vi "Panel Split Example.vi"(10 "Caller":string) -> ()   [LabVIEW 2013]
uses:
  PanelRootNode/PanelRootNode.lvclass
  <vilib>/Utility/error.llb/DialogType.ctl
  PanelExample.lvclass
  share/QueueManager.llb/Destroy.vi
  share/QueueManager.llb/CreatQueue.vi
  share/QueueManager.llb/Remove.vi
  PanelLinkNode/PanelLinkNode.lvclass
  PanelDataNode/PanelDataNode.lvclass
panel:
  out "SelfNode*":refnum<data-value>
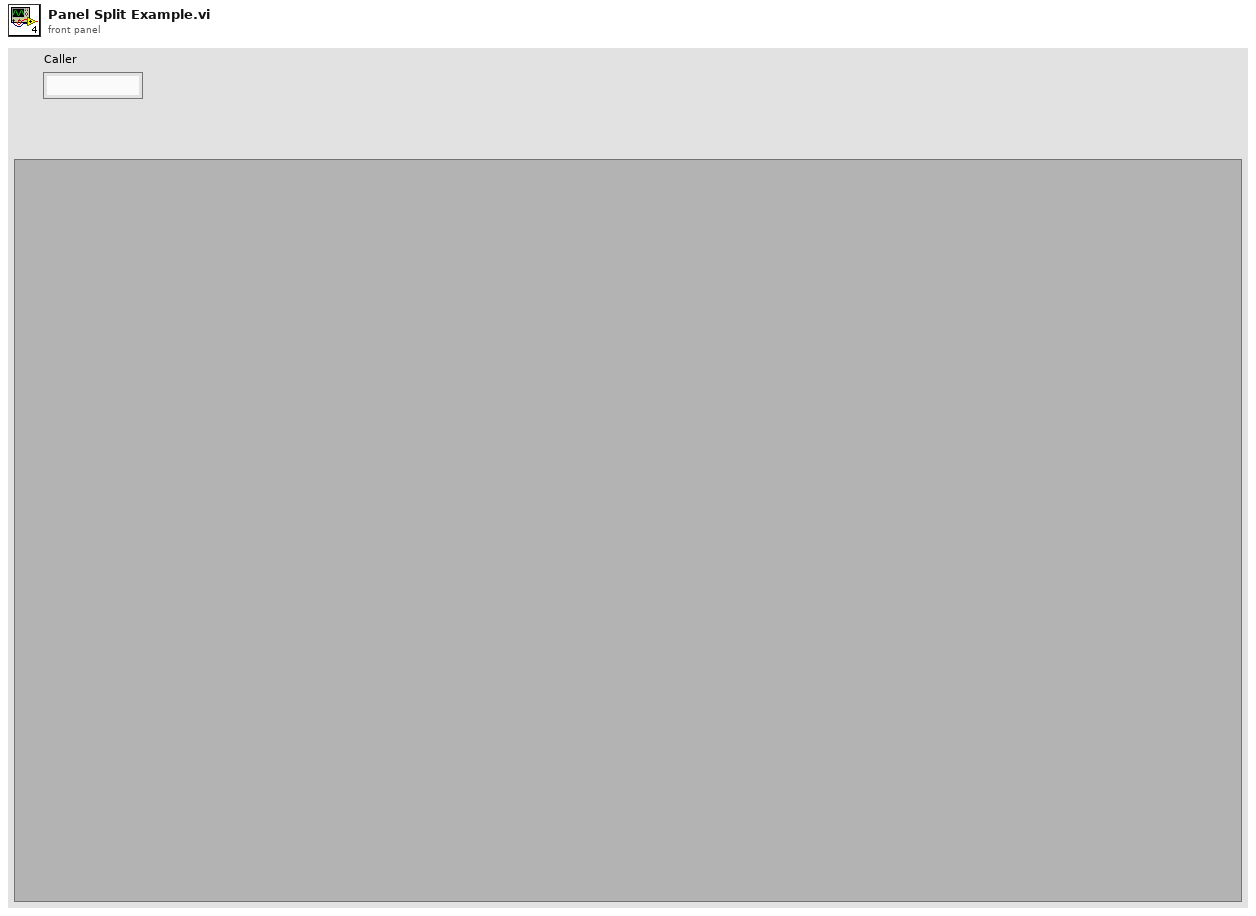
[diagram p1: front panel]
types:
  T1 = cluster{"error":errorcluster, "Event":string, "Data":variant, "Q_Local":string, "RootNode*":refnum<data-value>, "Caller":string}
  T2 = typedef "DialogType.ctl" = u16
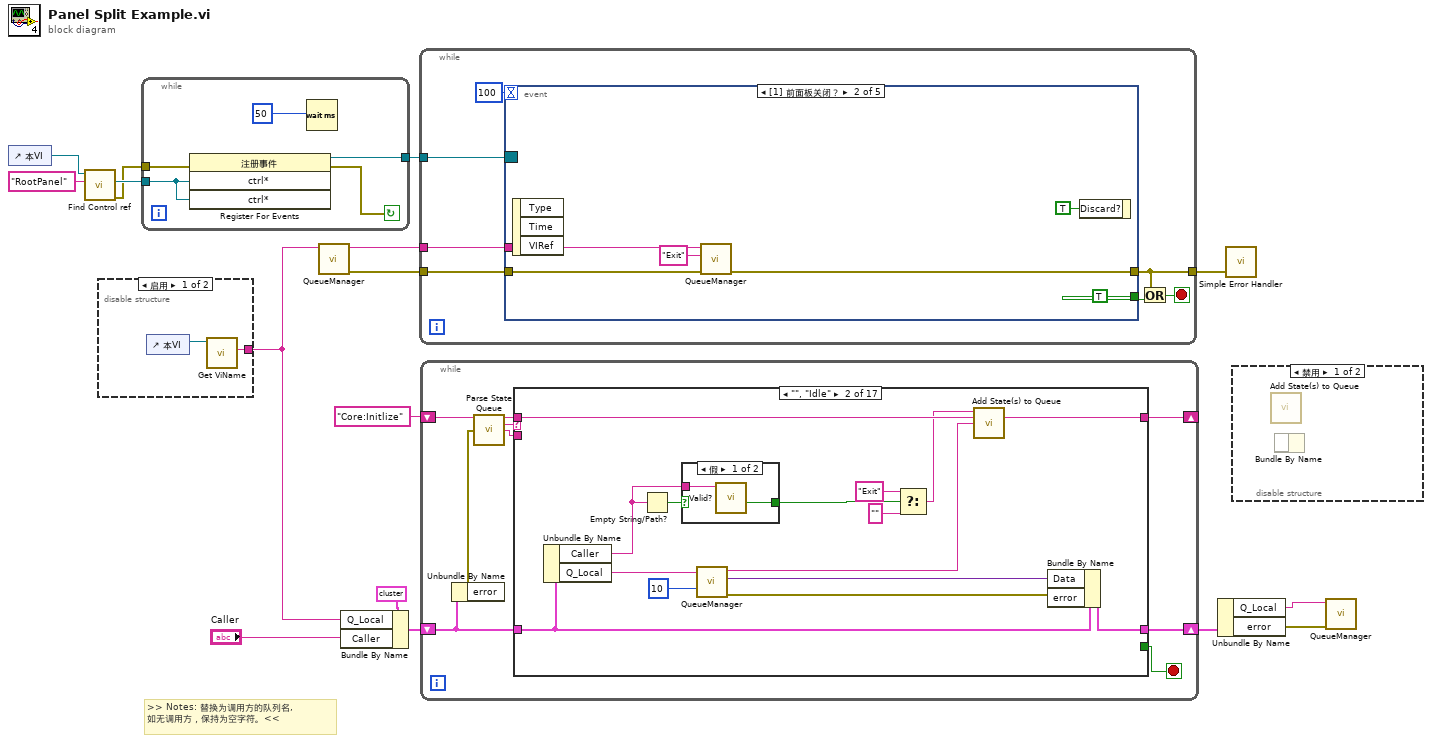
[diagram p0: block diagram]
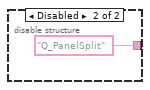
[diagram p2: hidden frame]
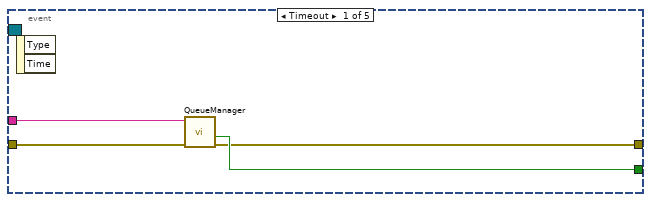
[diagram p4: hidden frame]
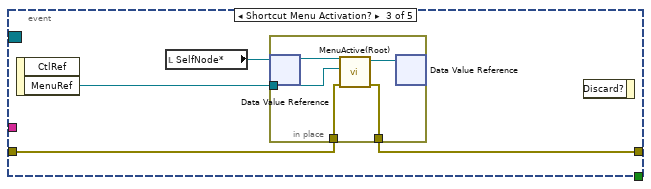
[diagram p5: hidden frame]
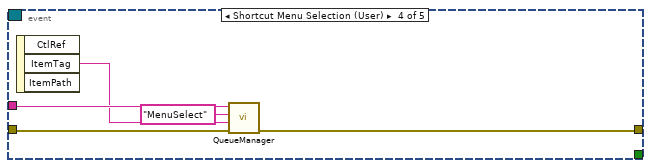
[diagram p6: hidden frame]
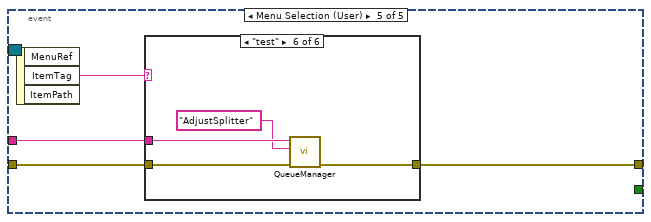
[diagram p7: hidden frame]
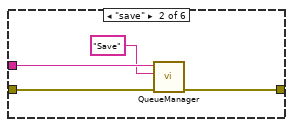
[diagram p9: hidden frame]
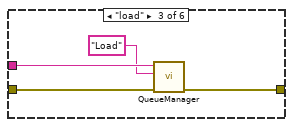
[diagram p10: hidden frame]
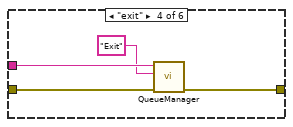
[diagram p11: hidden frame]
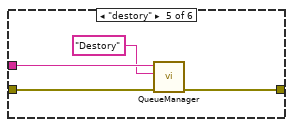
[diagram p12: hidden frame]
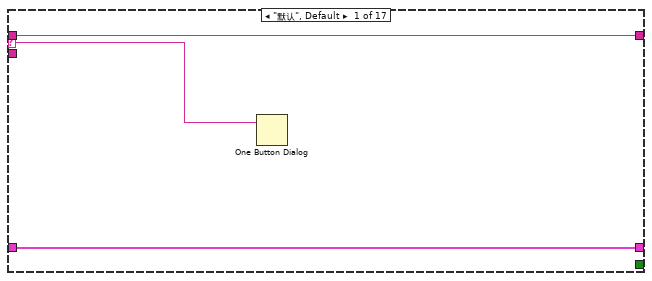
[diagram p13: hidden frame]
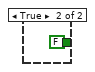
[diagram p14: hidden frame]
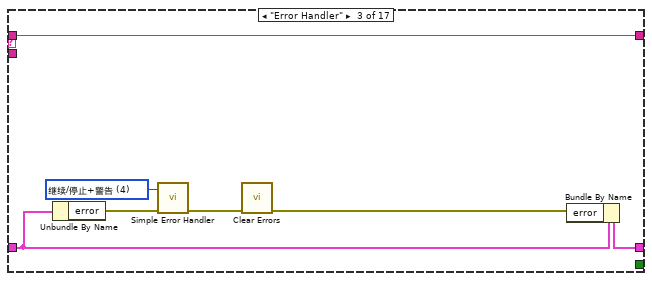
[diagram p15: hidden frame]
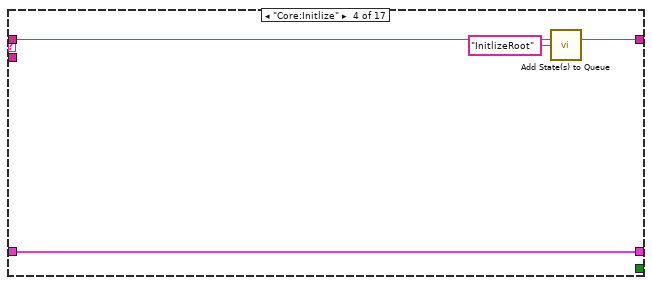
[diagram p16: hidden frame]
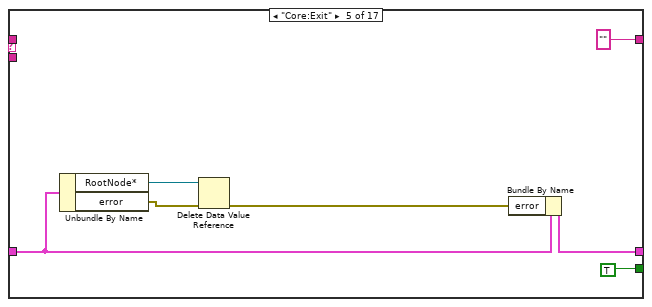
[diagram p17: hidden frame]
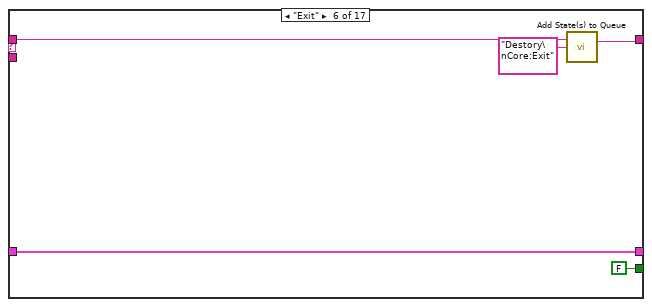
[diagram p18: hidden frame]
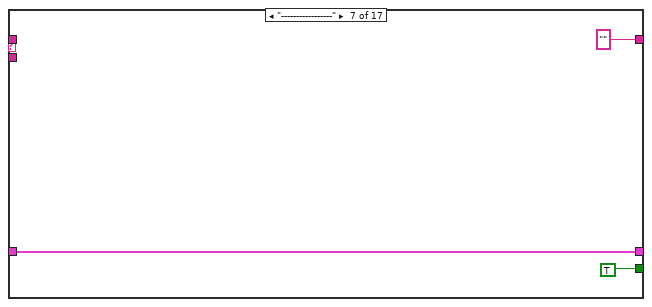
[diagram p19: hidden frame]
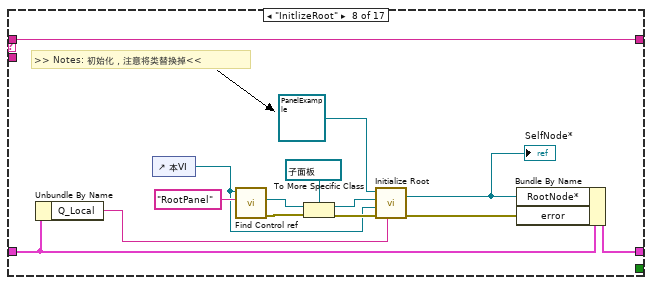
[diagram p20: hidden frame]
diagram:
  # ">> Notes: 替换为调用方的队列名,\n如无调用方，保持为空字符。<<"
  n1 = control-ref of="本VI"() -> (w7:refnum<vi>)
  n2 = call "Find Control ref.vi"("control name"="RootPanel", "panelvi*"=w7) -> ("error out"=w2:errorcluster, "ctrl*"=w5:refnum<vi>)  [unwired: 7 in, 1 out]
  n3 = disable-structure shown="启用" {
    disable-tunnel: [w16 "Q_PanelSplit" ("QueueName")] -> w3
    frame Enabled {
      n4 = control-ref of="本VI"() -> (w17:refnum<vi>)
      n5 = call "Get ViName.vi"("VI*"=w17) -> ("VI Name"=w16:string)  [unwired: 8 in, 2 out]
    }
    frame Disabled {
    }
  }
  n6 = while {
    tunnel: w5 -> [w23]
    tunnel: [w22] -> w4
    tunnel: w2 -> [w21]
    stop <- w20 continue-if-true
    n7 = register-events(error in=w21, w23, w23) -> (reference out=w22:refnum<event-registration>, error out=w20:errorcluster)  [unwired: 1 in]
    n8 = Wait (ms)(milliseconds to wait=50) -> ()  [unwired: 1 out]
  }
  n9 = call-poly "QueueManager.vi"("QueueName"=w3) -> ("error out"=w15:errorcluster)  [unwired: 10 in]
  n10 = Bundle By Name(cluster=T1 {"error"={"status"=FALSE, "code"=0, "source"=""}, "Event"="", "Data"=variant, "Q_Local"="", "RootNode*"=refnum, "Caller"=""} ("TmpData"), "Q_Local"=w3, "Caller"="Caller") -> (w9:T1)
  n11 = while {
    tunnel: w15 -> [w29]
    tunnel: w3 -> [w30]
    tunnel: [w26] -> w11
    tunnel: w4 -> [w24]
    stop <- w27 stop-if-true
    n12 = event shown="[1] 前面板关闭？" {
      selector: w24 -> [_ _ _ _ _]
      dyn-events: _ -> [_ _ _ _ _]
      timeout: 100 -> [_ _ _ _ _]
      tunnel: [w32 TRUE _ _ _] -> w28
      tunnel: w30 -> [w34 w39 _ w54 w57]
      tunnel: w29 -> [w33 w38 w43 w53 w56]
      tunnel: [w31 w37 w44 w52 w55] -> w26
      event Timeout {
        n13 = event-data() -> ()  [unwired: 1 in, 2 out]
        n14 = call-poly "QueueManager.vi"("error in (no error)"=w33, "Queue Name(unamed)"=w34) -> ("error out"=w31:errorcluster, "Not Exist?"=w32:bool)  [unwired: 8 in]
      }
      event Panel Close? {
        n15 = event-data() -> ()  [unwired: 1 in, 3 out]
        n16 = call-poly "QueueManager.vi"("error in"=w38, "Event"="Exit", "QueueName"=w39) -> ("error out"=w37:errorcluster)  [unwired: 7 in, 1 out]
        n17 = event-data("Discard?"=TRUE ("放弃？")) -> ()  [unwired: 1 in, 1 out]
      }
      event Shortcut Menu Activation? {
        n18 = event-data() -> ("MenuRef"=w42:refnum<k9>)  [unwired: 1 in, 1 out]
        n19 = local read "SelfNode*"() -> (w41:refnum<data-value>)
        n20 = in-place {
          in-place-border: w42 -> [w47]
          in-place-border: w43 -> [w46]
          in-place-border: [w45] -> w44
          n21 = in-place-dvr #1(w41) -> (w49:refnum<class "PanelRootNode.lvclass">)  [unwired: 1 out]
          n22 = call "MenuActive(Root).vi"("error in (no error)"=w46, "菜单引用"=w47, "PanelDataNode 输入"=w49) -> ("error out"=w45:errorcluster, "PanelDataNode 输出"=w48:refnum<class "PanelRootNode.lvclass">)  [unwired: 7 in]
          n23 = in-place-dvr #1(w48) -> ()  [unwired: 2 out]
        }
        n24 = event-data() -> ()  [unwired: 2 in, 1 out]
      }
      event Shortcut Menu Selection (User) {
        n25 = event-data() -> ("ItemTag"=w51:string)  [unwired: 1 in, 2 out]
        n26 = call-poly "QueueManager.vi"("error in"=w53, "Data"=w51, "Event"="MenuSelect", "QueueName"=w54) -> ("error out"=w52:errorcluster)  [unwired: 6 in, 1 out]
      }
      event Menu Selection (User) {
        n27 = event-data() -> ("ItemTag"=w58:string)  [unwired: 1 in, 2 out]
        n28 = case shown="\"test\"" w58 {
          tunnel: w57 -> [_ w63 w67 w71 w75 w79]
          tunnel: w56 -> [w59 w61 w65 w69 w73 w77]
          tunnel: [w59 w60 w64 w68 w72 w76] -> w55
          frame "假", Default {
          }
          frame "save" {
            n29 = call-poly "QueueManager.vi"("error in"=w61, "Event"="Save", "QueueName"=w63) -> ("error out"=w60:errorcluster)  [unwired: 7 in, 1 out]
          }
          frame "load" {
            n30 = call-poly "QueueManager.vi"("error in"=w65, "Event"="Load", "QueueName"=w67) -> ("error out"=w64:errorcluster)  [unwired: 7 in, 1 out]
          }
          frame "exit" {
            n31 = call-poly "QueueManager.vi"("error in"=w69, "Event"="Exit", "QueueName"=w71) -> ("error out"=w68:errorcluster)  [unwired: 7 in, 1 out]
          }
          frame "destory" {
            n32 = call-poly "QueueManager.vi"("error in"=w73, "Event"="Destory", "QueueName"=w75) -> ("error out"=w72:errorcluster)  [unwired: 7 in, 1 out]
          }
          frame "test" {
            n33 = call-poly "QueueManager.vi"("error in"=w77, "Event"="AdjustSplitter", "QueueName"=w79) -> ("error out"=w76:errorcluster)  [unwired: 7 in, 1 out]
          }
        }
      }
    }
    n34 = Or(x=w26, y=w28) -> (x .or. y?=w27:bool)
  }
  n35 = while {
    shift-right: [w81] -> w12
    shift-left: w9 -> [w82]
    shift-right: [w80] -> _
    shift-left: "Core:Initlize" -> [w88]
    stop <- w84 stop-if-true
    n36 = Unbundle By Name(w82) -> ("error"=w83:errorcluster)
    n37 = call "Parse State Queue.vi"("State Queue"=w88, "Error In (no error)"=w83) -> ("Remaining States"=w87:string, "Current State"=w86:string, "Arguments"=w85:string)  [unwired: 10 in, 1 out]
    n38 = case shown="\"\", \"Idle\"" w86 {
      selector: w86 -> [w89 _ _ _ _ _ _ _ _ _ _ _ _ _ _ _ _]
      tunnel: w87 -> [w90 w102 w116 w119 _ w132 _ w149 w155 w171 w181 w196 w206 w216 w226 w235 w250]
      tunnel: w85 -> [_ _ _ _ _ _ _ _ _ _ _ _ _ _ _ _ _]
      tunnel: [_ _ _ _ TRUE FALSE TRUE _ _ _ _ _ _ _ _ _ _] -> w84
      tunnel: w82 -> [w91 w99 w112 w120 w123 w129 w134 w138 w157 w169 w185 w195 w204 w214 w224 w233 w248]
      tunnel: [w91 w105 w111 w120 w122 w129 w134 w141 w156 w168 w184 w194 w203 w213 w223 w232 w247] -> w81
      tunnel: [w90 w101 w116 w118 "" ("Remaining States") w131 "" ("Remaining States") w149 w155 w171 w180 w196 w206 w216 w226 w235 w250] -> w80
      frame "默认", Default {
        n39 = One Button Dialog(message=w89) -> ()  [unwired: 1 in, 1 out]
      }
      frame "", "Idle" {
        n40 = Unbundle By Name(w99) -> ("Caller"=w93:string, "Q_Local"=w98:string)
        n41 = Empty String/Path?(string/path=w93) -> (empty?=w97:bool)
        n42 = case shown="假" w97 {
          tunnel: [w108 FALSE ("Not Exist?")] -> w96
          tunnel: w93 -> [w107 _]
          frame False {
            n43 = call "Valid?.vi"("Queue Name(unamed)"=w107) -> ("Not Exist?"=w108:bool)  [unwired: 9 in, 1 out]
          }
          frame True {
          }
        }
        n44 = call-poly "QueueManager.vi"("Time out(-1)"=10, "Queue Name"=w98) -> ("error out"=w106:errorcluster, "Data"=w104:variant, "Event"=w103:string)  [unwired: 6 in, 1 out]
        n45 = Select(t="Exit" ("Event"), s=w96, f="") -> (s? t:f=w92:string)
        n46 = call "Add State(s) to Queue.vi"("State(s) in Front (\"\")"=w92, "State(s) in (\"\")"=w102, "State(s) at Back (\"\")"=w103) -> ("States Out"=w101:string)  [unwired: 12 in]
        n47 = Bundle By Name(cluster=w99, "Data"=w104, "error"=w106) -> (w105:T1)
      }
      frame "Error Handler" {
        w110 = T2 4 items=["无对话框", "确定信息", "继续或停止信息", "确定信息＋警告", "继续/停止+警告"] ("type of dialog (OK msg:1)")
        n48 = Unbundle By Name(w112) -> ("error"=w113:errorcluster)
        n49 = call <vilib>:"Simple Error Handler.vi"("type of dialog (OK msg:1)"=w110, "error in (no error)"=w113) -> ("error out"=w114:errorcluster)  [unwired: 3 in, 4 out]
        n50 = call <vilib>:"Clear Errors.vi"("error in (no error)"=w114) -> ("error out"=w115:errorcluster)  [unwired: 6 in]
        n51 = Bundle By Name(cluster=w112, "error"=w115) -> (w111:T1)
      }
      frame "Core:Initlize" {
        n52 = call "Add State(s) to Queue.vi"("State(s) in (\"\")"=w119, "State(s) at Back (\"\")"="InitlizeRoot" ("State(s) at Back (\"\")")) -> ("States Out"=w118:string)  [unwired: 13 in]
      }
      frame "Core:Exit" {
        n53 = Unbundle By Name(w123) -> ("RootNode*"=w125:refnum<data-value>, "error"=w121:errorcluster)
        n54 = Delete Data Value Reference(data value reference=w125, error in=w121) -> (error out=w124:errorcluster)  [unwired: 1 out]
        n55 = Bundle By Name(cluster=w123, "error"=w124) -> (w122:T1)
      }
      frame "Exit" {
        n56 = call "Add State(s) to Queue.vi"("State(s) in (\"\")"=w132, "State(s) at Back (\"\")"="Destory\nCore:Exit" ("State(s) at Back (\"\")")) -> ("States Out"=w131:string)  [unwired: 13 in]
      }
      frame "-----------------" {
      }
      frame "InitlizeRoot" {
        # ">> Notes: 初始化，注意将类替换掉<<"
        n57 = Unbundle By Name(w138) -> ("Q_Local"=w137:string)
        n58 = control-ref of="本VI"() -> (w139:refnum<vi>)
        n59 = call "Find Control ref.vi"("control name"="RootPanel", "panelvi*"=w139) -> ("error out"=w144:errorcluster, "ctrl*"=w148:refnum<vi>)  [unwired: 7 in, 1 out]
        n60 = To More Specific Class(target class=refnum<vi> refnum ("RootPanel"), reference=w148, error in=w144) -> (specific class reference=w146:refnum<vi>, error out=w143:errorcluster)
        n61 = call-dynamic "Initialize Root.vi"("RootQueueName"=w137, "error in (no error)"=w143, "CurrentVi*"=w139, "RootPanel*"=w146, "PanelRootNode 输入"=refnum<class "PanelExample.lvclass"> refnum ("PanelExample.lvclass")) -> ("error out"=w142:errorcluster, "SelfNode*"=w140:refnum<data-value>)  [unwired: 5 in]
        "SelfNode*" <- w140
        n62 = Bundle By Name(cluster=w138, "RootNode*"=w140, "error"=w142) -> (w141:T1)
      }
      frame "Save" {
        # ">> Notes: 保存分割结果<<"
        n63 = Unbundle By Name(w157) -> ("RootNode*"=w158:refnum<data-value>, "Data"=w153:variant)
        n64 = Variant To Data(type=path "" ("路径"), Variant=w153) -> (data=w151:path, error out=w150:errorcluster)  [unwired: 1 in]
        n65 = call <vilib>:"Clear Errors.vi"("error in (no error)"=w150) -> ()  [unwired: 6 in, 1 out]
        n66 = in-place {
          in-place-border: [w160] -> w154
          in-place-border: w151 -> [w159]
          n67 = in-place-dvr #2(w158) -> (w162:refnum<class "PanelRootNode.lvclass">)  [unwired: 1 out]
          n68 = call-dynamic "Save Xml.vi"("selected path"=w159, "PanelRootNode 输入"=w162) -> ("error out"=w160:errorcluster, "PanelRootNode 输出"=w161:refnum<class "PanelRootNode.lvclass">)  [unwired: 8 in]
          n69 = in-place-dvr #2(w161) -> ()  [unwired: 2 out]
        }
        n70 = Bundle By Name(cluster=w157, "error"=w154) -> (w156:T1)
      }
      frame "Load" {
        n71 = Unbundle By Name(w169) -> ("RootNode*"=w170:refnum<data-value>, "Data"=w164:variant)
        n72 = Variant To Data(type=path "" ("路径"), Variant=w164) -> (data=w163:path, error out=w165:errorcluster)  [unwired: 1 in]
        n73 = call <vilib>:"Clear Errors.vi"("error in (no error)"=w165) -> ()  [unwired: 6 in, 1 out]
        n74 = in-place {
          in-place-border: [w174] -> w167
          in-place-border: w163 -> [w172]
          n75 = in-place-dvr #3(w170) -> (w173:refnum<class "PanelRootNode.lvclass">)  [unwired: 1 out]
          n76 = call-dynamic "Load Xml.vi"("selected path"=w172, "PanelRootNode 输入"=w173) -> ("error out"=w174:errorcluster, "PanelRootNode 输出"=w175:refnum<class "PanelRootNode.lvclass">)  [unwired: 8 in]
          n77 = in-place-dvr #3(w175) -> ()  [unwired: 2 out]
        }
        n78 = Bundle By Name(cluster=w169, "error"=w167) -> (w168:T1)
      }
      frame "MenuSelect" {
        n79 = Unbundle By Name(w185) -> ("RootNode*"=w179:refnum<data-value>, "Data"=w183:variant)
        n80 = Variant To Data(type="", Variant=w183) -> (data=w178:string, error out=w177:errorcluster)  [unwired: 1 in]
        n81 = in-place {
          in-place-border: w178 -> [w188]
          in-place-border: w177 -> [w187]
          in-place-border: [w186] -> w176
          n82 = in-place-dvr #4(w179) -> (w190:refnum<class "PanelRootNode.lvclass">)  [unwired: 1 out]
          n83 = call-dynamic "MenuSelect.vi"("error in"=w187, "Tag"=w188, "PanelRootNode 输入"=w190) -> ("error out"=w186:errorcluster, "PanelRootNode 输出"=w189:refnum<class "PanelRootNode.lvclass">)  [unwired: 7 in]
          n84 = in-place-dvr #4(w189) -> ()  [unwired: 2 out]
        }
        n85 = Bundle By Name(cluster=w185, "error"=w176) -> (w184:T1)
        n86 = call "Add State(s) to Queue.vi"("State(s) in (\"\")"=w181) -> ("States Out"=w180:string)  [unwired: 14 in]
      }
      frame "Split" {
        n87 = Unbundle By Name(w195) -> ("RootNode*"=w193:refnum<data-value>, "Data"=w192:variant)
        n88 = in-place {
          in-place-border: w192 -> [w198]
          in-place-border: [w197] -> w191
          n89 = in-place-dvr #5(w193) -> (w200:refnum<class "PanelRootNode.lvclass">)  [unwired: 1 out]
          n90 = call-dynamic "Split.vi"("Data"=w198, "PanelRootNode 输入"=w200) -> ("error out"=w197:errorcluster, "PanelRootNode 输出"=w199:refnum<class "PanelRootNode.lvclass">)  [unwired: 8 in]
          n91 = in-place-dvr #5(w199) -> ()  [unwired: 2 out]
        }
        n92 = Bundle By Name(cluster=w195, "error"=w191) -> (w194:T1)
      }
      frame "Delete" {
        n93 = Unbundle By Name(w204) -> ("RootNode*"=w205:refnum<data-value>, "Data"=w202:variant)
        n94 = in-place {
          in-place-border: w202 -> [w208]
          in-place-border: [w207] -> w201
          n95 = in-place-dvr #6(w205) -> (w210:refnum<class "PanelRootNode.lvclass">)  [unwired: 1 out]
          n96 = call-dynamic "Delete.vi"("Data"=w208, "PanelRootNode 输入"=w210) -> ("error out"=w207:errorcluster, "PanelRootNode 输出"=w209:refnum<class "PanelRootNode.lvclass">)  [unwired: 8 in]
          n97 = in-place-dvr #6(w209) -> ()  [unwired: 2 out]
        }
        n98 = Bundle By Name(cluster=w204, "error"=w201) -> (w203:T1)
      }
      frame "Insert" {
        n99 = Unbundle By Name(w214) -> ("RootNode*"=w215:refnum<data-value>, "Data"=w211:variant)
        n100 = in-place {
          in-place-border: [w217] -> w212
          in-place-border: w211 -> [w218]
          n101 = in-place-dvr #7(w215) -> (w220:refnum<class "PanelRootNode.lvclass">)  [unwired: 1 out]
          n102 = call-dynamic "Insert.vi"("Data"=w218, "PanelRootNode 输入"=w220) -> ("error out"=w217:errorcluster, "PanelRootNode 输出"=w219:refnum<class "PanelRootNode.lvclass">)  [unwired: 8 in]
          n103 = in-place-dvr #7(w219) -> ()  [unwired: 2 out]
        }
        n104 = Bundle By Name(cluster=w214, "error"=w212) -> (w213:T1)
      }
      frame "Destory" {
        # ">> Notes: 销毁分割结果，回到最初状态<<"
        n105 = Unbundle By Name(w224) -> ("RootNode*"=w225:refnum<data-value>, "Data"=w222:variant)
        n106 = in-place {
          in-place-border: w222 -> [_]
          in-place-border: [w227] -> w221
          n107 = in-place-dvr #8(w225) -> (w229:refnum<class "PanelRootNode.lvclass">)  [unwired: 1 out]
          n108 = call-dynamic "Destory.vi"("PanelRootNode 输入"=w229) -> ("error out"=w227:errorcluster, "PanelRootNode 输出"=w228:refnum<class "PanelRootNode.lvclass">)  [unwired: 9 in]
          n109 = in-place-dvr #8(w228) -> ()  [unwired: 2 out]
        }
        n110 = Bundle By Name(cluster=w224, "error"=w221) -> (w223:T1)
      }
      frame "AdjustSplitter" {
        # ">> Notes: 均分面板<<"
        n111 = Unbundle By Name(w233) -> ("RootNode*"=w234:refnum<data-value>, "Data"=w231:variant)
        n112 = in-place {
          in-place-border: w231 -> [_]
          in-place-border: [w236] -> w230
          n113 = in-place-dvr #9(w234) -> (w238:refnum<class "PanelRootNode.lvclass">)  [unwired: 1 out]
          n114 = call "Adjust Splitter.vi"("PanelRootNode 输入"=w238) -> ("error out"=w236:errorcluster, "PanelRootNode 输出"=w237:refnum<class "PanelRootNode.lvclass">)  [unwired: 9 in]
          n115 = in-place-dvr #9(w237) -> ()  [unwired: 2 out]
        }
        n116 = Bundle By Name(cluster=w233, "error"=w230) -> (w232:T1)
      }
      frame "SendToAll" {
        # ">> Notes: 发送至所有面板中插入的VI线程，要求插入的VI使用的队列名是VI名称；<<"
        n117 = Unbundle By Name(w248) -> ("RootNode*"=w249:refnum<data-value>, "Data"=w245:variant, "error"=w239:errorcluster)
        n118 = Variant To Data(error in=w239, type=cluster{"Event":string, "Data":variant} {"Event"="", "Data"=variant}, Variant=w245) -> (data=w243:cluster{"Event":string, "Data":variant}, error out=w240:errorcluster)
        n119 = Unbundle By Name(w243) -> ("Event"=w242:string, "Data"=w241:variant)
        n120 = in-place {
          in-place-border: [w255] -> w246
          in-place-border: w242 -> [w254]
          in-place-border: w241 -> [w253]
          in-place-border: w240 -> [w252]
          n121 = in-place-dvr #10(w249) -> (w257:refnum<class "PanelRootNode.lvclass">)  [unwired: 1 out]
          n122 = call "SendToPanels.vi"("PanelNumber(-1)"=-1, "error in"=w252, "Data"=w253, "Event"=w254, "PanelRootNode 输入"=w257) -> ("error out"=w255:errorcluster, "PanelRootNode 输出"=w256:refnum<class "PanelRootNode.lvclass">)  [unwired: 5 in]
          n123 = in-place-dvr #10(w256) -> ()  [unwired: 2 out]
        }
        n124 = Bundle By Name(cluster=w248, "error"=w246) -> (w247:T1)
      }
    }
  }
  n125 = Unbundle By Name(w12) -> ("Q_Local"=w8:string, "error"=w13:errorcluster)
  n126 = call <vilib>:"Simple Error Handler.vi"("error in (no error)"=w11) -> ()  [unwired: 4 in, 5 out]
  n127 = disable-structure shown="禁用" {
    frame Disabled {
      n128 = call "Add State(s) to Queue.vi"() -> ()  [unwired: 15 in, 1 out]
      n129 = Bundle By Name() -> ()  [unwired: 2 in, 1 out]
    }
    frame Enabled {
    }
  }
  n130 = call-poly "QueueManager.vi"("error in (no error)"=w13, "QueeuName"=w8) -> ()  [unwired: 9 in, 1 out]
